vi "Search Key-Value-Pair by Key.vi"(8 "error in (no error)":errorcluster, 10 "Key":string, 11 "Key-Value-Pair List":T1[](array[typedef])) -> (0 "error out":errorcluster, 2 "Value":string, 3 "Key-Value-Pair List Passthrough":T1[](array[typedef]))   [LabVIEW 2011, in "i3-oauth.lvlib"]
uses:
  i3-oauth.lvlib
  key-value-pairs.ctl
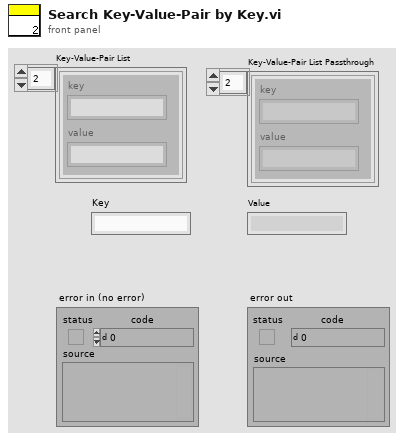
[diagram p1: front panel]
types:
  T1 = typedef "i3-oauth.lvlib/key-value-pairs.ctl" = cluster{"key":string, "value":string}
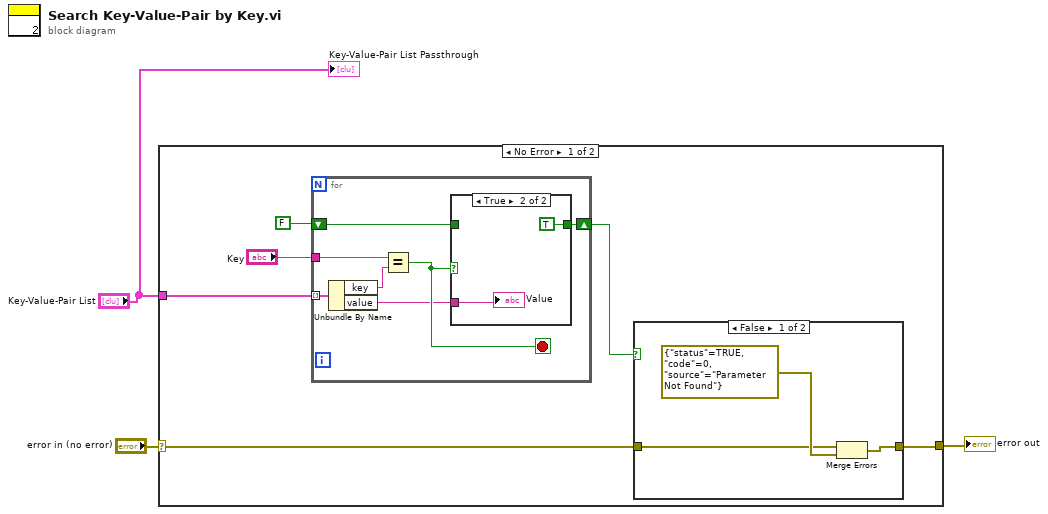
[diagram p0: block diagram]
diagram:
  n1 = case shown="No Error" "error in (no error)" {
    selector: "error in (no error)" -> [w6 w24]
    tunnel: [w5 w24] -> w2
    tunnel: "Key-Value-Pair List" -> [w4 _]
    frame No Error {
      n2 = for {
        tunnel: w4 -> [w20] mode=indexing
        tunnel: "Key" -> [w18]
        shift-right: [w14] -> w7
        shift-left: FALSE -> [w15]
        stop <- w17 stop-if-true
        n3 = Unbundle By Name(w20) -> ("key"=w19:string, "value"=w16:string)
        n4 = Equal?(x=w18, y=w19) -> (x = y?=w17:bool)
        n5 = case shown="True" w17 {
          tunnel: w16 -> [_ w23]
          tunnel: w15 -> [w21 _]
          tunnel: [w21 TRUE] -> w14
          frame False {
          }
          frame True {
            "Value" <- w23
          }
        }
      }
      n6 = case shown="False" w7 {
        tunnel: w6 -> [w11 w13]
        tunnel: [w10 w13] -> w5
        frame False {
          n7 = Merge Errors(w11, errorcluster {"status"=TRUE, "code"=0, "source"="Parameter Not Found"} ("error out")) -> (w10:errorcluster)
        }
        frame True {
        }
      }
    }
    frame Error {
    }
  }
  "error out" <- w2
  "Key-Value-Pair List Passthrough" <- "Key-Value-Pair List"
